vi "templates table HEADER data keys.vi"(9 "Template Keys":T1, 10 "HTM Keys":T1) -> (2 "HTM Keys":T1)   [LabVIEW 2011]
uses:
  Addons/internet/utils/keyedarr.llb/Keyed Array.ctl
  Addons/internet/utils/strutil.llb/Case Matching.ctl
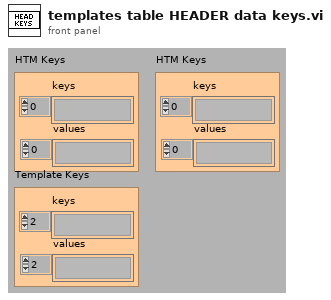
[diagram p1: front panel]
types:
  T1 = typedef "Keyed Array.ctl" = cluster{"keys":string[], "values":string[]}
  T2 = typedef "Case Matching.ctl" = enum16{"a != A", "a == A", "system"}
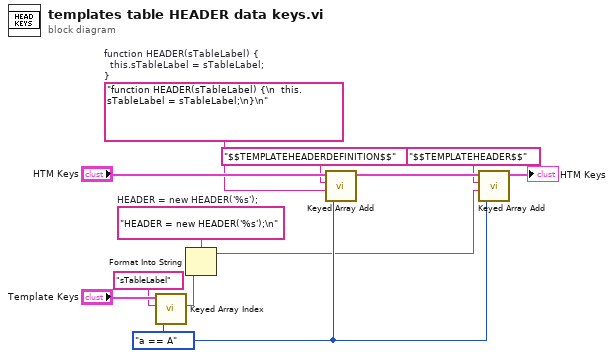
[diagram p0: block diagram]
diagram:
  w6 = "HEADER = new HEADER('%s');\n"  # HEADER = new HEADER('%s');
  w4 = Case_Matching."a == A" ("case matching (sensitive)")
  w10 = "function HEADER(sTableLabel) {\n  this.sTableLabel = sTableLabel;\n}\n"  # function HEADER(sTableLabel) {   this.sTableLabel = sTableLabel; }
  n1 = call "Keyed Array Index.vi"("case matching (sensitive)"=w4, "key"="sTableLabel", "array in"="Template Keys") -> ("value"=w1:string)  [unwired: 1 in, 3 out]
  n2 = Format Into String(format string=w6, w1) -> (resulting string=w3:string)  [unwired: 2 in, 1 out]
  n3 = call "Keyed Array Add.vi"("case matching (sensitive)"=w4, "value"=w10, "key"="$$TEMPLATEHEADERDEFINITION$$", "array in"="HTM Keys") -> ("array out"=w9:T1)  [unwired: 3 out]
  n4 = call "Keyed Array Add.vi"("case matching (sensitive)"=w4, "value"=w3, "key"="$$TEMPLATEHEADER$$", "array in"=w9) -> ("array out"=→"HTM Keys":T1)  [unwired: 3 out]
